vi "Create CSV.vi"(8 "error in (no error)":errorcluster, 10 "dma blocks":T1(array[cluster]), 11 "path":path) -> (0 "error out":errorcluster)   [LabVIEW 2017]
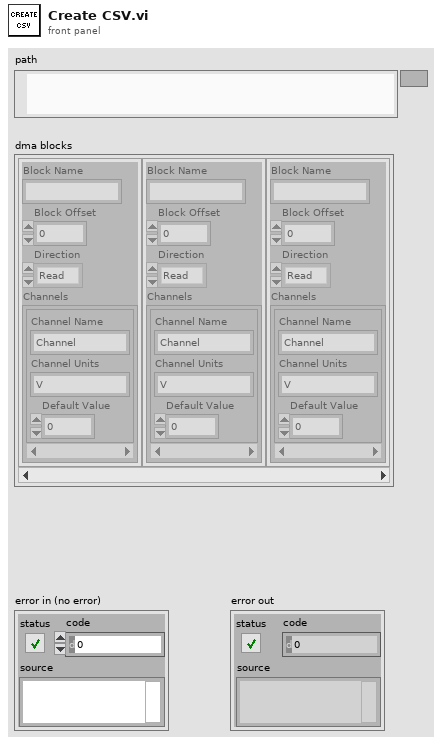
[diagram p1: front panel]
types:
  T1 = cluster{"Block Name":string, "Block Offset":u32, "Direction":enum16{"Read", "Write"}, "Channels":cluster{"Channel Name":string, "Channel Units":string, "Default Value":dbl}[]}[]
  T2 = enum16{"open", "replace", "create", "open or create", "replace or create", "replace or create with confirmation"}
  T3 = cluster{"Channel Name":string, "Channel Units":string, "Default Value":dbl}[]
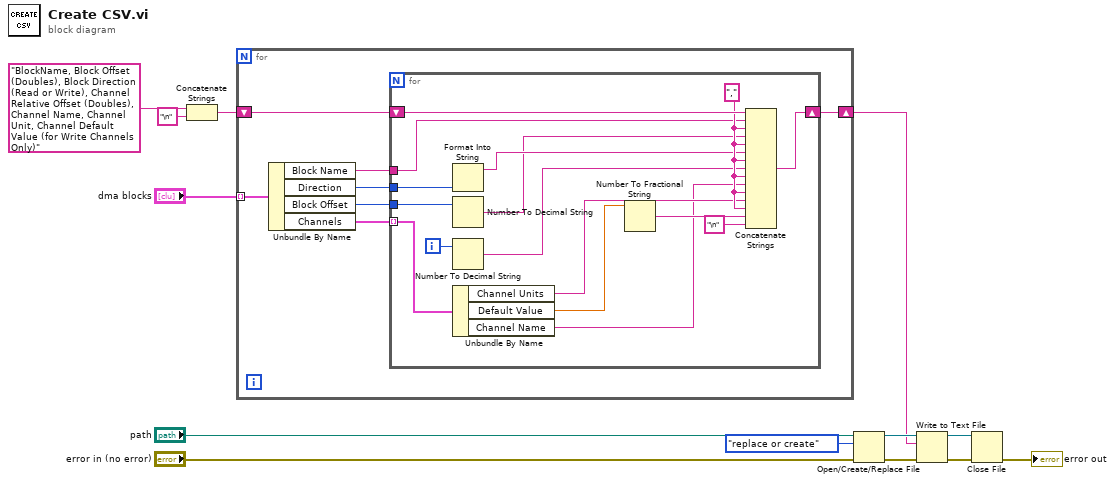
[diagram p0: block diagram]
diagram:
  n1 = Concatenate Strings("BlockName, Block Offset (Doubles), Block Direction (Read or Write), Channel Relative Offset (Doubles), Channel Name, Channel Unit, Channel Default Value (for Write Channels Only)", "\n" ("string")) -> (w4:string)
  n2 = for {
    tunnel: "dma blocks" -> [w20] mode=indexing
    shift-right: [w18] -> w3
    shift-left: w4 -> [w19]
    n3 = Unbundle By Name(w20) -> ("Block Name"=w15:string, "Direction"=w14:enum16{"Read", "Write"}, "Block Offset"=w17:u32, "Channels"=w16:T3)
    n4 = for {
      shift-right: [w35] -> w18
      shift-left: w19 -> [w36]
      tunnel: w17 -> [w33]
      tunnel: w15 -> [w29]
      tunnel: w16 -> [w34] mode=indexing
      tunnel: w14 -> [w23]
      i -> [w27]
      w31 = ","
      n5 = Format Into String(w23) -> (resulting string=w30:string)  [unwired: 3 in, 1 out]
      n6 = Number To Decimal String(number=w33) -> (decimal integer string=w28:string)  [unwired: 1 in]
      n7 = Number To Decimal String(number=w27) -> (decimal integer string=w26:string)  [unwired: 1 in]
      n8 = Unbundle By Name(w34) -> ("Channel Units"=w25:string, "Default Value"=w32:dbl, "Channel Name"=w21:string)
      n9 = Number To Fractional String(number=w32) -> (F-format string=w24:string)  [unwired: 3 in]
      n10 = Concatenate Strings(w36, w29, w31, w28, w31, w30, w31, w26, w31, w21, w31, w25, w31, w24, "\n" ("string")) -> (w35:string)
    }
  }
  n11 = Open/Create/Replace File(file path (use dialog)="path", error in="error in (no error)", operation (0:open)=T2."replace or create") -> (refnum out=w11:refnum<file>, error out=w10:errorcluster)  [unwired: 3 in, 1 out]
  n12 = Write to Text File(file (use dialog)=w11, text=w3, error in=w10) -> (refnum out=w8:refnum<file>, error out=w9:errorcluster)  [unwired: 1 in, 1 out]
  n13 = Close File(refnum=w8, error in=w9) -> (error out=→"error out":errorcluster)  [unwired: 1 out]
